vi "Initialize Dialog.vi"(8 "error in (no error)":errorcluster, 9 "dialog options in":T1={"angle mode"=1, "picture pixels per unit"=30.0, "close window on exit"=FALSE, "window behavior"=enum."Default"} {"angle mode" items=["Degrees", "Radians"]}, 10 "FP Refs":T5, 11 "steering frame ref in":refnum<data-value>) -> (0 "error out":errorcluster, 2 "subpanel to main command event reg":T3, 3 "dialog info":T4={"steering frame ref"=refnum, "active wheel indexes"=[], "FP Refs"={"VI Refnum"=refnum, "Menu Ref"=refnum, "Sub Panel"=refnum, "picture"=refnum, "Steering Type"=refnum, "zoom in"=refnum, "zoom out"=refnum, "zoom extents"=refnum, "Wheels"=refnum, "Add Wheel"=refnum, "Remove Wheel"=refnum, "Copy Wheel"=refnum, "Angle Units"=refnum}, "subpanel info"={"subpanel VI refs"=[], "subpanel types"=[], "main to subpanel command events"=[]}, "picture dragging state"={"dragging"=FALSE, "wheel index"=-1, "dragging mode"=enum."translate", "wheel start position"={"x"=0.0, "y"=0.0, "theta"=0.0}, "relative mouse position"={"x"=0.0, "y"=0.0}, "relative mouse init angle (rad)"=0.0}, "picture size (pixels)"={"Width"=500, "Height"=500}, "picture grid"=bytes[0], "click zones group"={"click zones array"=[], "num click zones"=0}, "draw options"={"draw wheel states?"=FALSE, "highlight wheel index"=-1, "pixels per unit"=10.0, "draw forward velocity?"=FALSE, "velocity scale"=1.0}})   [LabVIEW 2017, in "NI_Robotics_Configure Steering Frame.lvlib"]
uses:
  <vilib>/robotics/Dialog/Configure Steering Frame/NI_Robotics_Configure Steering Frame.lvlib
  <vilib>/robotics/Dialog/Configure Steering Frame/FP Refs.ctl
  <vilib>/robotics/Dialog/Configure Steering Frame/Dialog Info.ctl
  <vilib>/robotics/Steering/Steering Frame/NI_Robotics_Steering Frame.lvclass
  <vilib>/robotics/Dialog/Configure Steering Frame/Subpanel Info.ctl
  <vilib>/robotics/Dialog/Configure Steering Frame/Main to Subpanel Command Event.ctl
  <vilib>/robotics/Dialog/Configure Steering Frame/Main to Subpanel Command.ctl
  <vilib>/robotics/Dialog/Configure Steering Frame/Dragging State.ctl
  <vilib>/robotics/Dialog/Configure Steering Frame/Dragging Mode.ctl
  <vilib>/Utility/miscctls.llb/LVBoundsTypeDef.ctl
  <vilib>/robotics/Dialog/Configure Steering Frame/Click Zone.ctl
  <vilib>/robotics/Utilities/Visualization/Steering Visualization/Steering Picture/Draw Steering Frame Options.ctl
  <vilib>/robotics/Dialog/Configure Steering Frame/Subpanel to Main Command Event Reg.ctl
  <vilib>/robotics/Dialog/Configure Steering Frame/Dialog Options.ctl
  <vilib>/robotics/Dialog/Configure Steering Frame/Angle Mode.ctl
  <vilib>/robotics/Steering/Steering Frame/NI_Robotics_Steering Frame.lvclass/NI_Robotics_Steering Frame.ctl
  <vilib>/robotics/Utilities/Generate Error.vi
  <vilib>/robotics/Utilities/Visualization/Steering Visualization/Steering Picture/NI_Robotics_Steering Picture.lvlib
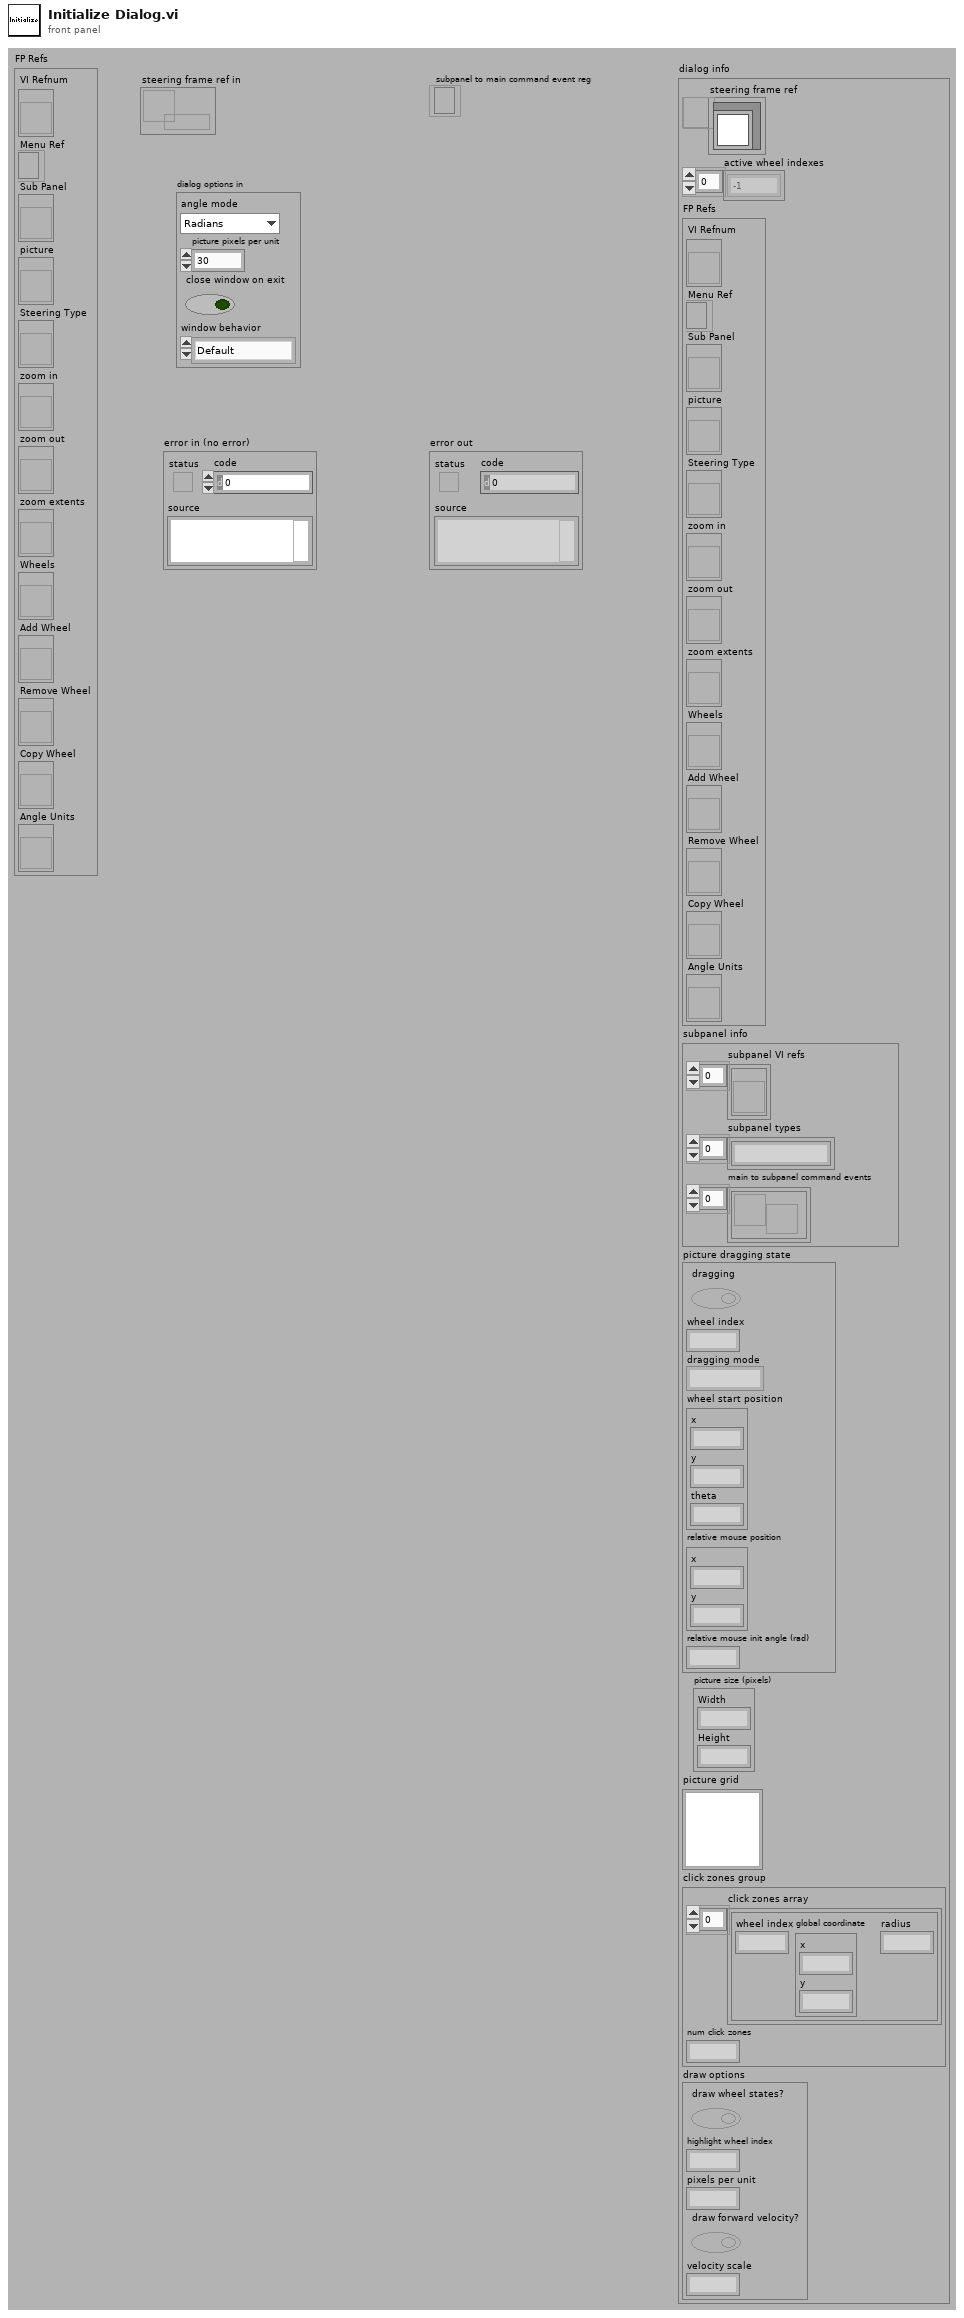
[diagram p1: front panel]
types:
  T1 = typedef "NI_Robotics_Configure Steering Frame.lvlib/Dialog Options.ctl" = cluster{"angle mode":T2, "picture pixels per unit":dbl, "close window on exit":bool, "window behavior":enum32{"Invalid", "Default", "Floating", "Floating/Auto-Hide", "Modal"}}
  T2 = typedef "NI_Robotics_Configure Steering Frame.lvlib/Angle Mode.ctl" = u16
  T3 = typedef "NI_Robotics_Configure Steering Frame.lvlib/Subpanel to Main Command Event Reg.ctl" = refnum<event-registration>
  T4 = typedef "NI_Robotics_Configure Steering Frame.lvlib/Dialog Info.ctl" = cluster{"steering frame ref":refnum<data-value>, "active wheel indexes":i32[], "FP Refs":T5, "subpanel info":T6, "picture dragging state":T8, "picture size (pixels)":T10, "picture grid":picture, "click zones group":cluster{"click zones array":T11[], "num click zones":i32}, "draw options":T12}
  T5 = typedef "NI_Robotics_Configure Steering Frame.lvlib/FP Refs.ctl" = cluster{"VI Refnum":refnum<vi>, "Menu Ref":refnum<k9>, "Sub Panel":refnum<vi>, "picture":refnum<vi>, "Steering Type":refnum<vi>, "zoom in":refnum<vi>, "zoom out":refnum<vi>, "zoom extents":refnum<vi>, "Wheels":refnum<vi>, "Add Wheel":refnum<vi>, "Remove Wheel":refnum<vi>, "Copy Wheel":refnum<vi>, "Angle Units":refnum<vi>}
  T6 = typedef "NI_Robotics_Configure Steering Frame.lvlib/Subpanel Info.ctl" = cluster{"subpanel VI refs":refnum<vi>[], "subpanel types":string[], "main to subpanel command events":T7[]}
  T7 = typedef "NI_Robotics_Configure Steering Frame.lvlib/Main to Subpanel Command Event.ctl" = refnum<user-event>
  T8 = typedef "NI_Robotics_Configure Steering Frame.lvlib/Dragging State.ctl" = cluster{"dragging":bool, "wheel index":i32, "dragging mode":T9, "wheel start position":cluster{"x":dbl, "y":dbl, "theta":dbl}, "relative mouse position":cluster{"x":dbl, "y":dbl}, "relative mouse init angle (rad)":dbl}
  T9 = typedef "NI_Robotics_Configure Steering Frame.lvlib/Dragging Mode.ctl" = enum16{"translate", "rotate"}
  T10 = typedef "LVBoundsTypeDef.ctl" = cluster{"Width":u32, "Height":u32}
  T11 = typedef "NI_Robotics_Configure Steering Frame.lvlib/Click Zone.ctl" = cluster{"wheel index":i32, "global coordinate":cluster{"x":dbl, "y":dbl}, "radius":dbl}
  T12 = typedef "NI_Robotics_Steering Picture.lvlib/Draw Steering Frame Options.ctl" = cluster{"draw wheel states?":bool, "highlight wheel index":i32, "pixels per unit":dbl, "draw forward velocity?":bool, "velocity scale":dbl}
  T13 = enum32{"Invalid", "Default", "Floating", "Floating/Auto-Hide", "Modal"}
  T14 = cluster{"elements":T11[], "number of elements":i32}
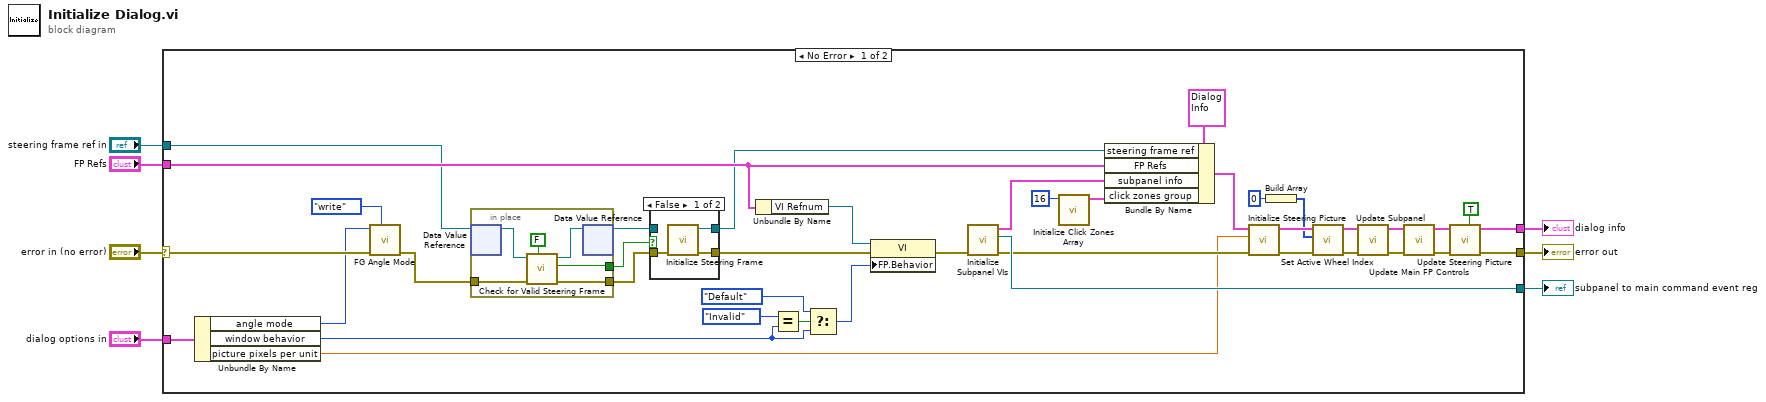
[diagram p0: block diagram]
diagram:
  n1 = case shown="No Error" "error in (no error)" {
    selector: "error in (no error)" -> [w47 w59]
    tunnel: "FP Refs" -> [w43 _]
    tunnel: [w40 w59] -> w5
    tunnel: [w45 _] -> w4
    tunnel: [w28 _] -> w3
    tunnel: "steering frame ref in" -> [w34 _]
    tunnel: "dialog options in" -> [w32 _]
    frame No Error {
      n2 = Unbundle By Name(w32) -> ("angle mode"=w31:T2, "window behavior"=w12:T13, "picture pixels per unit"=w19:dbl)
      n3 = call <vilib>:"FG Angle Mode.vi"("action (read)"=enum16{"read", "write"}."write", "error in (no error)"=w47, "angle mode in"=w31) -> ("error out"=w23:errorcluster)  [unwired: 7 in, 1 out]
      n4 = in-place {
        in-place-border: [w51] -> w36
        in-place-border: w23 -> [w50]
        in-place-border: [w49] -> w35
        n5 = in-place-dvr #1(w34) -> (w53:refnum<class "NI_Robotics_Steering Frame.lvclass">)  [unwired: 1 out]
        n6 = call <vilib>:"Check for Valid Steering Frame.vi"("produce error if invalid (T)"=FALSE, "error in (no error)"=w50, "steering frame in"=w53) -> ("error out"=w51:errorcluster, "valid?"=w49:bool, "steering frame out"=w52:refnum<class "NI_Robotics_Steering Frame.lvclass">)  [unwired: 6 in]
        n7 = in-place-dvr #1(w52) -> (w33:refnum<data-value>)  [unwired: 1 out]
      }
      n8 = case shown="False" w35 {
        tunnel: [w56 w58] -> w39
        tunnel: w36 -> [w55 w57]
        tunnel: [w54 w57] -> w16
        tunnel: w33 -> [_ w58]
        frame False {
          n9 = call <vilib>:"Initialize Steering Frame.vi"("error in (no error)"=w55) -> ("error out"=w54:errorcluster, "steering frame"=w56:refnum<data-value>)  [unwired: 9 in]
        }
        frame True {
        }
      }
      n10 = Unbundle By Name(w43) -> ("VI Refnum"=w18:refnum<vi>)
      n11 = Equal?(x=T13."Invalid", y=w12) -> (x = y?=w14:bool)
      n12 = Select(t=T13."Default" ("x"), s=w14, f=w12) -> (s? t:f=w11:T13)
      n13 = property class="VI"(reference=w18, error in=w16, "FP.Behavior"=w11) -> (error out=w17:errorcluster)  [unwired: 1 out]
      n14 = call <vilib>:"Initialize Subpanel VIs.vi"("error in (no error)"=w17) -> ("error out"=w29:errorcluster, "subpanel to main command event reg"=w45:T3, "subpanel info"=w44:T6)  [unwired: 8 in]
      n15 = call <vilib>:"Initialize Click Zones Array.vi"("size"=16) -> ("array"=w20:T14)  [unwired: 10 in]
      n16 = Bundle By Name(cluster=T4 {"steering frame ref"=refnum, "active wheel indexes"=[], "FP Refs"={"VI Refnum"=refnum, "Menu Ref"=refnum, "Sub Panel"=refnum, "picture"=refnum, "Steering Type"=refnum, "zoom in"=refnum, "zoom out"=refnum, "zoom extents"=refnum, "Wheels"=refnum, "Add Wheel"=refnum, "Remove Wheel"=refnum, "Copy Wheel"=refnum, "Angle Units"=refnum}, "subpanel info"={"subpanel VI refs"=[], "subpanel types"=[], "main to subpanel command events"=[]}, "picture dragging state"={"dragging"=FALSE, "wheel index"=0, "dragging mode"=enum."translate", "wheel start position"={"x"=0.0, "y"=0.0, "theta"=0.0}, "relative mouse position"={"x"=0.0, "y"=0.0}, "relative mouse init angle (rad)"=0.0}, "picture size (pixels)"={"Width"=0, "Height"=0}, "picture grid"=bytes[0], "click zones group"={"click zones array"=[], "num click zones"=0}, "draw options"={"draw wheel states?"=FALSE, "highlight wheel index"=0, "pixels per unit"=0.0, "draw forward velocity?"=FALSE, "velocity scale"=0.0}} ("dialog info"), "steering frame ref"=w39, "FP Refs"=w43, "subpanel info"=w44, "click zones group"=w20) -> (w30:T4)
      n17 = call <vilib>:"Initialize Steering Picture.vi"("error in (no error)"=w29, "pixels per unit"=w19, "dialog info in"=w30) -> ("error out"=w25:errorcluster, "dialog info out"=w27:T4)  [unwired: 7 in]
      n18 = Build Array(0 ("active wheel index")) -> (w8:i32[])
      n19 = call <vilib>:"Set Active Wheel Index.vi"("error in (no error)"=w25, "active wheel indexes"=w8, "dialog info in"=w27) -> ("error out"=w24:errorcluster, "dialog info out"=w26:T4)  [unwired: 7 in]
      n20 = call <vilib>:"Update Subpanel.vi"("error in (no error)"=w24, "dialog info in"=w26) -> ("error out"=w37:errorcluster, "dialog info out"=w38:T4)  [unwired: 8 in]
      n21 = call <vilib>:"Update Main FP Controls.vi"("error in (no error)"=w37, "dialog info in"=w38) -> ("error out"=w41:errorcluster, "dialog info out"=w42:T4)  [unwired: 8 in]
      n22 = call <vilib>:"Update Steering Picture.vi"("redraw grid (F)"=TRUE, "error in (no error)"=w41, "dialog info in"=w42) -> ("error out"=w40:errorcluster, "dialog info out"=w28:T4)  [unwired: 7 in]
    }
    frame Error {
    }
  }
  "error out" <- w5
  "dialog info" <- w3
  "subpanel to main command event reg" <- w4
